vi "Initialize.vi"(8 "error in (no error)":errorcluster, 11 "NhRegenGridSim in":refnum<class "NHRGridSim.lvclass">) -> (0 "error out":errorcluster, 3 "NhRegenGridSim out":refnum<class "NHRGridSim.lvclass">)   [LabVIEW 2018, in "AcPwrPlugins.lvlib" / "NHRGridSim.lvclass"]
doc: "This VI opens a connection to the instrument(s). It optionally resets the instrument or checks that the phase ID is valid."
uses:
  NHRGridSim.lvclass
  <instrlib>/NH Research 9400 Series/NH Research 9400 Series.lvlib
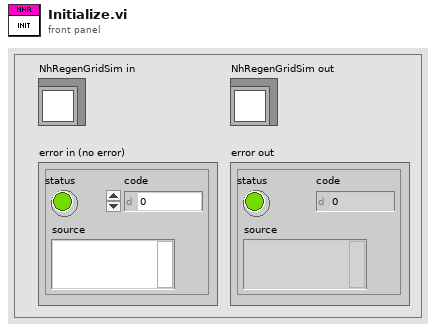
[diagram p1: front panel]
types:
  T1 = cluster{"Boolean":bool, "VISA Resource":refnum<visa-resource-name>}
  T2 = typedef "AcPwrPlugins.lvlib/NHRGridSim.lvclass/Device(s)Settings.ctl" = cluster{"MeasName":string, "Instr1":T3, "Instr2":T3, "Instr3":T3, "Handle":string, "Reset":bool, "Mode":T9, "ID Query":bool, "Connected":bool, "Chassis":i32, "VRangeVals1":string[], "SyncList1":string[], "Wave1A":string[], "Wave1B":string[], "Wave1C":string[], "SyncList2":string[], "SyncList3":string[], "VRangeVals3":string[], "VRangeVals2":string[], "CRangeVals1":string[], "CRangeVals3":string[], "CRangeVals2":string[], "TabPages":bool[], "Wave2A":string[], "Wave2B":string[], "Wave2C":string[], "Wave3A":string[], "Wave3B":string[], "Wave3C":string[], "EnableCtrls":i8[][]}
  T3 = typedef "AcPwrPlugins.lvlib/NHRGridSim.lvclass/NHRGrid_InstrumentCluster_Tabs.ctl" = cluster{"Name":string, "Vout (V)":dbl, "VType":string, "FreqOut (Hz)":dbl, "Aperture (cycles)":i32, "Synchronization":T4, "Ranges":T5, "Safety Trips":T6, "Slew Rates":T7, "Phases":T8}
  T4 = typedef "AcPwrPlugins.lvlib/NHRGridSim.lvclass/NHRGrid_Configure_Tabs.ctl" = u16
  T5 = typedef "AcPwrPlugins.lvlib/NHRGridSim.lvclass/NHRGrid_Ranges_Tabs.ctl" = cluster{"Voltage (V)":u16, "Current (A)":u16}
  T6 = typedef "AcPwrPlugins.lvlib/NHRGridSim.lvclass/NHRGrid_SafetyTrips_Tabs.ctl" = cluster{"Vmin (V)":dbl, "Vmin Time (s)":dbl, "Vmax (V)":dbl, "Vmax Time (s)":dbl, "Imax Source (A)":dbl, "I Src Time (s)":dbl, "Imax Sink (A)":dbl, "I Snk Time (s)":dbl, "Pmax Source (W)":dbl, "P Src Time (s)":dbl, "Pmax Sink (W)":dbl, "P Snk Time (s)":dbl, "Abs Volt Peak":dbl, "Enable Vpk":bool, "Abs Curr Peak":dbl, "Enable Ipk":bool}
  T7 = typedef "AcPwrPlugins.lvlib/NHRGridSim.lvclass/NHRGrid_SlewRates_Tabs.ctl" = cluster{"Voltage (V/s)":dbl, "Current (A/s)":dbl, "Power (W/s)":dbl, "Frequency (Hz/s)":dbl, "Phase Angle (Deg/s)":dbl}
  T8 = typedef "AcPwrPlugins.lvlib/NHRGridSim.lvclass/NHRGrid_Phases_Tabs.ctl" = cluster{"A-Volts (V)":dbl, "B-Volts (V)":dbl, "C-Volts (V)":dbl, "A-Change at...":i32, "B-Angle (Deg)":i32, "C-Angle (Deg)":i32, "B-Change at...":i32, "C-Change at...":i32, "AngleTxt":string, "A-Wave Shape":u16, "B-Wave Shape":u16, "C-Wave Shape":u16}
  T9 = typedef "AcPwrPlugins.lvlib/NHRGridSim.lvclass/NHRGrid_Modes.ctl" = u8
  T10 = typedef "AcPwrPlugins.lvlib/NHRGridSim.lvclass/Measurements.ctl" = cluster{"Handle":string, "Name":string, "Enabled ":bool, "Measurement Value":dbl, "Instrument Number ":i32, "Measurement Type ":T11}[]
  T11 = typedef "AcPwrPlugins.lvlib/NHRGridSim.lvclass/MeasurementType.ctl" = enum16{"Average Current", "Average Voltage"}
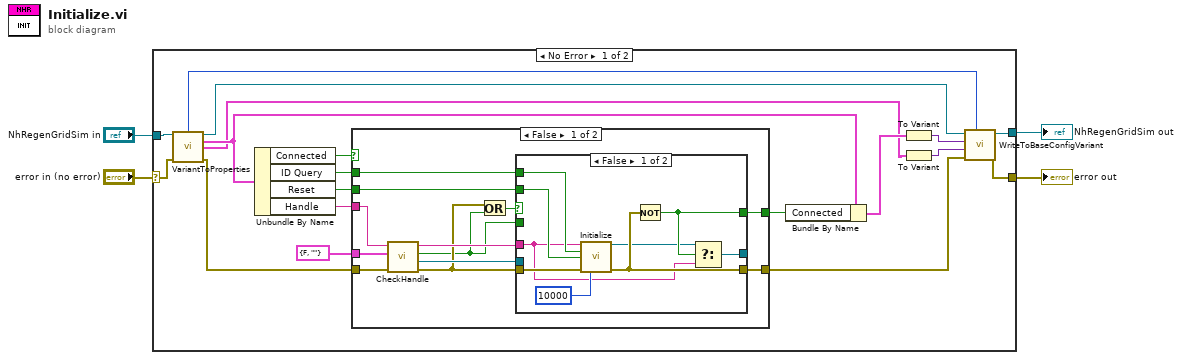
[diagram p0: block diagram]
diagram:
  n1 = case shown="No Error" "error in (no error)" {
    selector: "error in (no error)" -> [w22 w50]
    tunnel: "NhRegenGridSim in" -> [w23 w51]
    tunnel: [w18 w51] -> w2
    tunnel: [w17 w50] -> w1
    frame No Error {
      n2 = call "VariantToProperties.vi"("NHRGridSim in"=w23, "error in (no error)"=w22) -> ("NHRGridSim out"=w19:refnum<class "NHRGridSim.lvclass">, "Device(s)Settings"=w7:T2, "Measurements"=w5:T10, "Measurement Refresh Time (ms)"=w14:u32, "error out"=w21:errorcluster)  [unwired: 8 in, 1 out]
      n3 = Unbundle By Name(w7) -> ("Connected"=w13:bool, "ID Query"=w12:bool, "Reset"=w11:bool, "Handle"=w10:string)
      n4 = case shown="False" w13 {
        selector: w13 -> [_ w48]
        tunnel: w21 -> [w31 w49]
        tunnel: [w33 w49] -> w16
        tunnel: w11 -> [w35 _]
        tunnel: w12 -> [w34 _]
        tunnel: w10 -> [w30 _]
        tunnel: [w32 w48] -> w9
        tunnel: T1 {"Boolean"=FALSE, "VISA Resource"=""} ("Resource In") -> [w24 _]
        frame False {
          n5 = call "CheckHandle.vi"("Error In"=w31, "Resource In"=w24, "Handle In"=w30) -> ("Error Out"=w26:errorcluster, "VISA Resource"=w28:refnum<visa-resource-name>, "Handle Connected?"=w25:bool, "Handle Out"=w29:string)  [unwired: 5 in]
          n6 = Or(x=w26, y=w25) -> (x .or. y?=w27:bool)
          n7 = case shown="False" w27 {
            tunnel: w26 -> [w44 w47]
            tunnel: w35 -> [w43 _]
            tunnel: w34 -> [w42 _]
            tunnel: w29 -> [w36 _]
            tunnel: [w41 w47] -> w33
            tunnel: [w40 w45] -> w32
            tunnel: [w38 w46] -> _
            tunnel: w28 -> [_ w46]
            tunnel: w25 -> [_ w45]
            frame False {
              n8 = call <instrlib>:"Initialize.vi"("VISA resource name"=w36, "ID Query (True)"=w42, "Reset (True)"=w43, "error in (no error)"=w44, "Timeout (10000 ms)"=u32 10000) -> ("VISA resource name out"=w39:refnum<visa-resource-name>, "error out"=w41:errorcluster)  [unwired: 9 in]
              n9 = Not(x=w41) -> (.not. x?=w40:bool)
              n10 = Select(t=w39, s=w40, f=w36) -> (s? t:f=w38:refnum<visa-resource-name>)
            }
            frame True {
            }
          }
        }
        frame True {
        }
      }
      n11 = Bundle By Name(cluster=w7, "Connected"=w9) -> (w6:T2)
      n12 = To Variant(anything=w6) -> (Variant=w20:variant)
      n13 = To Variant(anything=w5) -> (Variant=w15:variant)
      n14 = call-dynamic "WriteToBaseConfigVariant.vi"("Measurement RefreshTime (ms)"=w14, "error in (no error)"=w16, "Meas"=w15, "Config"=w20, "NHRGridSim in"=w19) -> ("error out"=w17:errorcluster, "NHRGridSim out"=w18:refnum<class "NHRGridSim.lvclass">)  [unwired: 5 in]
    }
    frame Error {
    }
  }
  "error out" <- w1
  "NhRegenGridSim out" <- w2
